vi "VSTest - Deploy and Run SLSC Module.vi"(8 "error in (no error)":errorcluster, 9 "Gateway IP Address":string="localhost", 10 "Slot Module Number":u32=3, 11 "SLSC Chassis IP Address":string="10.2.228.104") -> (0 "error out":errorcluster, 3 "Passed?":bool)   [LabVIEW 2015, in "SLSC EDS Testing.lvlib"]
uses:
  SLSC EDS Testing.lvlib
  <vilib>/Utility/sysdir.llb/System Directory Type.ctl
  <vilib>/NI Veristand/Execution/Workspace/NI VeriStand - Get Multiple Channel Values.vi
  <vilib>/NI Veristand/Execution/Workspace/NI_VS Workspace ExecutionAPI.lvlib
  SLSC UI API/SLSC Tree Control.lvlib
  SLSC EDS API/SLSC EDS API.lvlib
panel:
  out "Command to launch VS":string
  out "appended path":path
  out "State":string="Done!"
  out "Initial State Defined?":bool
  out "Dynamic Property Equal?":bool
  out "Measured Values":dbl[](array[numeric])=[3.0, 5.0]
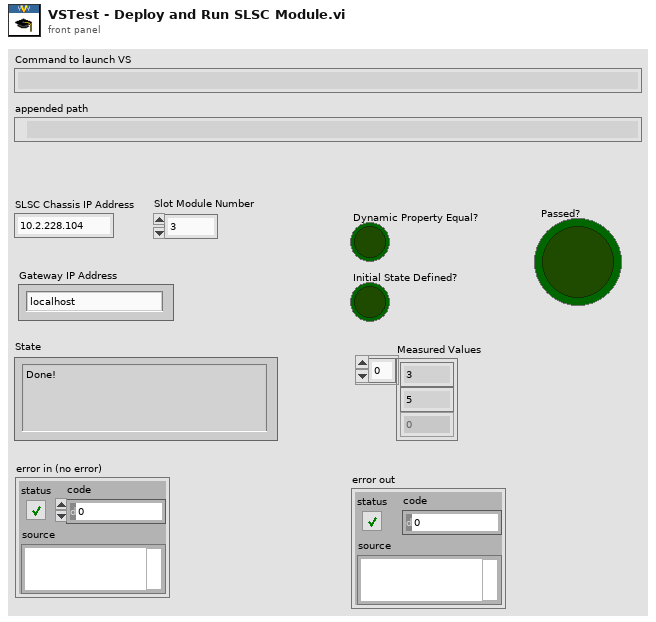
[diagram p1: front panel]
types:
  T1 = typedef "System Directory Type.ctl" = i32
  T2 = typedef "EDSjsonStructure.ctl" = cluster{"vendorNum":u32, "vendorName":string, "vendorPrefix":string, "productNum":u32, "productName":string, "capsVersion":string, "capsSpecVersion":u32, "capsSpecOldestCompatibleVersion":u32, "enums":T3[], "properties":T4[], "commands":T5[], "scales":T6[], "physicalChannels":T7[], "registerMap":cluster{"registers":T8[]}}
  T3 = typedef "enum.ctl" = cluster{"name":string, "description-en":string, "values":cluster{"name":string, "description-en":string, "value":i32}[]}
  T4 = typedef "property.ctl" = cluster{"name":string, "description-en":string, "documentation-en":string, "dataType":string, "bitfield":string, "access":string, "scale":string, "value":variant, "min":variant, "max":variant, "default value":variant}
  T5 = typedef "command.ctl" = cluster{"name":string, "description-en":string, "documentation-en":string, "startBitfield":string, "waitTimeInMs":i32, "doneBitfield":string, "doneInterrupt":string, "doneTimeoutInMs":i32, "value":variant}
  T6 = typedef "scale.ctl" = cluster{"name":string, "description-en":string, "m":dbl, "b":dbl, "forwardCoeffs":dbl[], "reverseCoeffs":dbl[], "coercion":string, "table":cluster{"scaled":dbl, "unscaled":dbl}[]}
  T7 = typedef "physicalChannel.ctl" = cluster{"name":string, "description-en":string, "commands":T5[], "properties":T4[]}
  T8 = typedef "register.ctl" = cluster{"name":string, "description-en":string, "access":string, "address":u32, "size":u32, "bitfields":cluster{"name":string, "description-en":string, "offset":u32, "size":u32, "signed":bool, "strobe":bool}[]}
  T9 = typedef "NI_VS Workspace ExecutionAPI.lvlib/WorkspaceAPI.ctl" = refnum<k24>
  T10 = cluster{"Left Cell String":string, "Child Text":string[], "Child Tag":string, "Item Indent":i32, "Child Only?":bool, "Glyph Index":i32}[]
  T11 = cluster{"Left Cell String":string, "Child Text":string[], "Child Tag":string, "Item Indent":i32, "Child Only?":bool, "Glyph Index":i32}
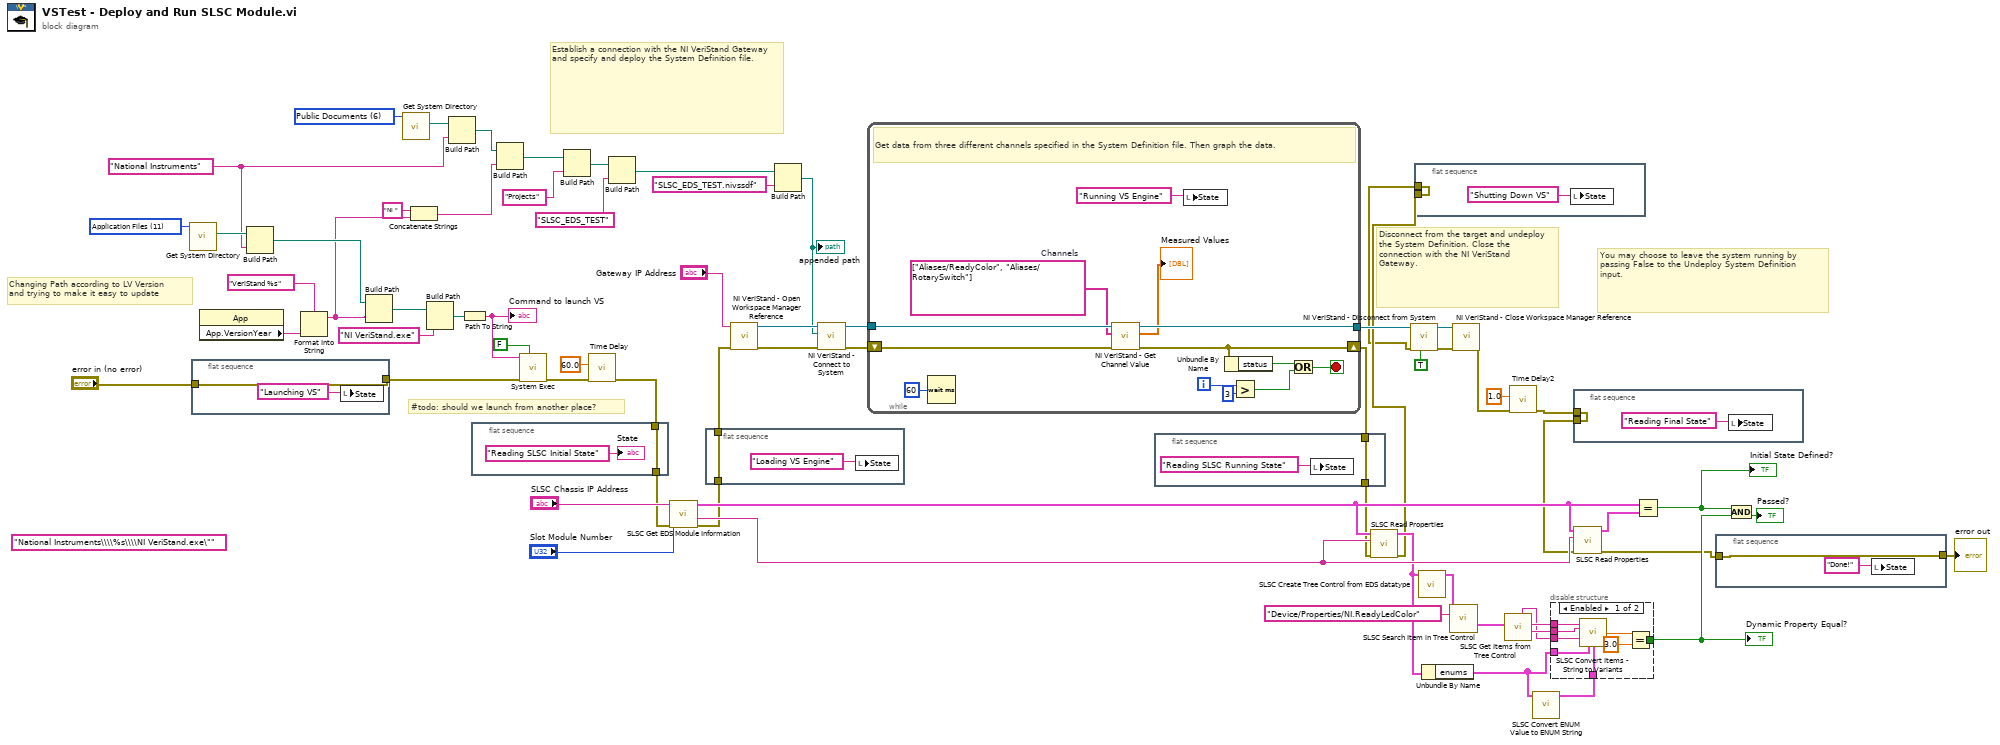
[diagram p0: block diagram]
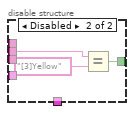
[diagram p2: hidden frame]
diagram:
  w15 = "National Instruments" ("command line")
  w20 = T1 11 items=["User Home"=0, "User Desktop"=1, "User Documents"=2, "User Application Data"=3, "User Preferences"=4, "User Temporary"=5, "Public Documents"=6, "Public Application Data"=7, "Public Preferences"=8, "Public Cache"=13, "System Core Libraries"=9, "System Installed Libraries"=10, "Application Files"=11, "Boot Volume Root"=12] ("system directory type")
  w21 = T1 6 items=["User Home"=0, "User Desktop"=1, "User Documents"=2, "User Application Data"=3, "User Preferences"=4, "User Temporary"=5, "Public Documents"=6, "Public Application Data"=7, "Public Preferences"=8, "Public Cache"=13, "System Core Libraries"=9, "System Installed Libraries"=10, "Application Files"=11, "Boot Volume Root"=12] ("system directory type")
  (unwired) "National Instruments\\\\%s\\\\NI VeriStand.exe\"" ("command line")
  # "Changing Path according to LV Version\nand trying to make it easy to update"
  # "#todo: should we launch from another place?"
  # "You may choose to leave the system running by passing False to the Undeploy System Definition input."
  # "Establish a connection with the NI VeriStand Gateway and specify and deploy the System Definition file."
  # "Disconnect from the target and undeploy the System Definition. Close the connection with the NI VeriStand Gateway."
  n1 = call <vilib>:"Get System Directory.vi"("system directory type"=w20) -> ("system directory"=w16:path)  [unwired: 10 in]
  n2 = flat-sequence {
    tunnel: "error in (no error)" -> [w69]
    tunnel: [w69] -> w23
    frame #0 {
      n3 = local write "State"("Launching VS" ("State")) -> ()
    }
  }
  n4 = property class="App"() -> ("App.VersionYear"=w22:string)  [unwired: 2 in, 2 out]
  n5 = Build Path(base path=w16, name or relative path=w15) -> (appended path=w14:path)
  n6 = Format Into String(format string="VeriStand %s" ("command line"), w22) -> (resulting string=w13:string)  [unwired: 2 in, 1 out]
  n7 = Build Path(base path=w14, name or relative path=w13) -> (appended path=w8:path)
  n8 = call <vilib>:"Get System Directory.vi"("system directory type"=w21) -> ("system directory"=w19:path)  [unwired: 10 in]
  n9 = Concatenate Strings("NI " ("string"), w13) -> (w3:string)
  n10 = Build Path(base path=w8, name or relative path="NI VeriStand.exe" ("command line")) -> (appended path=w7:path)
  n11 = Build Path(base path=w19, name or relative path=w15) -> (appended path=w17:path)
  n12 = Path To String(path=w7) -> (string=w10:string)
  "Command to launch VS" <- w10
  n13 = flat-sequence {
    tunnel: w35 -> [w71]
    tunnel: [w71] -> w34
    frame #0 {
      "State" <- "Reading SLSC Initial State" ("State")
    }
  }
  n14 = Build Path(base path=w17, name or relative path=w3) -> (appended path=w6:path)
  n15 = call <vilib>:"System Exec.vi"("wait until completion? (T)"=FALSE, "error in (no error)"=w23, "command line"=w10) -> ("error out"=w59:errorcluster)  [unwired: 5 in, 3 out]
  n16 = Build Path(base path=w6, name or relative path="Projects") -> (appended path=w5:path)
  n17 = call "Time Delay"("error in (no error)"=w59, "Delay Time (s)"=60.0) -> ("error out"=w35:errorcluster)  [unwired: 9 in]
  n18 = Build Path(base path=w5, name or relative path="SLSC_EDS_TEST") -> (appended path=w12:path)
  n19 = call "SLSC Get EDS Module Information.vi"("error in (no error)"=w34, "Slot #"="Slot Module Number", "Chassis IP Address"="SLSC Chassis IP Address") -> ("error out"=w33:errorcluster, "SLSC Module Name"=w41:string, "SLSC EDS module"=w42:T2)  [unwired: 5 in, 1 out]
  n20 = flat-sequence {
    tunnel: w33 -> [w73]
    tunnel: [w73] -> w32
    frame #0 {
      n21 = local write "State"("Loading VS Engine" ("State")) -> ()
    }
  }
  n22 = call <vilib>:"NI VeriStand - Open Workspace Manager Reference.vi"("error in (no error)"=w32, "Gateway IP Address (\"\": localhost)"="Gateway IP Address") -> ("error out"=w61:errorcluster, "WorkspaceManager"=w60:T9)  [unwired: 8 in]
  n23 = Build Path(base path=w12, name or relative path="SLSC_EDS_TEST.nivssdf") -> (appended path=w51:path)
  "appended path" <- w51
  n24 = call <vilib>:"NI VeriStand - Connect to System.vi"("error in (no error)"=w61, "System Definition File (.nivssdf)"=w51, "WorkspaceManager in"=w60) -> ("error out"=w64:errorcluster, "WorkspaceManager out"=w63:T9)  [unwired: 7 in]
  n25 = while {
    shift-right: [w84] -> w31
    shift-left: w64 -> [w85]
    tunnel: w63 -> [w83]
    tunnel: [w82] -> w62
    i -> [w78]
    stop <- w87 stop-if-true
    w80 = string[] ["Aliases/ReadyColor", "Aliases/RotarySwitch"]  # Channels
    # "Get data from three different channels specified in the System Definition file. Then graph the data."
    n26 = Wait (ms)(milliseconds to wait=u32 60) -> ()  [unwired: 1 out]
    n27 = call-poly <vilib>:"NI VeriStand - Get Channel Value.vi"("error in (no error)"=w85, "Channels"=w80, "WorkspaceManager in"=w83) -> ("error out"=w84:errorcluster, "Values"=→"Measured Values":dbl[], "WorkspaceManager out"=w82:T9)  [unwired: 6 in]
    n28 = local write "State"("Running VS Engine" ("State")) -> ()
    n29 = Unbundle By Name(w84) -> ("status"=w86:bool)
    n30 = Greater?(x=w78, y=3) -> (0:w76:bool)
    n31 = Or(x=w86, y=w76) -> (x .or. y?=w87:bool)
  }
  n32 = flat-sequence {
    tunnel: w31 -> [w88]
    tunnel: [w88] -> w30
    frame #0 {
      n33 = local write "State"("Reading SLSC Running State" ("State")) -> ()
    }
  }
  n34 = call "SLSC Read Properties.vi"("error in (no error)"=w30, "SLSC Device"=w41, "SLSC EDS module in"=w42) -> ("error out"=w29:errorcluster, "SLSC EDS module out"=w38:T2)  [unwired: 7 in]
  n35 = call <vilib>:"NI VeriStand - Disconnect from System.vi"("Undeploy System Definition (F)"=TRUE, "error in (no error)"=w28, "WorkspaceManager in"=w62) -> ("error out"=w67:errorcluster, "WorkspaceManager out"=w66:T9)  [unwired: 7 in]
  n36 = flat-sequence {
    tunnel: w29 -> [w90]
    tunnel: [w90] -> w28
    frame #0 {
      n37 = local write "State"("Shutting Down VS" ("State")) -> ()
    }
  }
  n38 = call "SLSC Create Tree Control from EDS datatype.vi"("SLSC EDS module"=w38) -> ("SLSC Output Tree"=w39:T10)  [unwired: 7 in, 3 out]
  n39 = Unbundle By Name(w38) -> ("enums"=w37:T3[])
  n40 = call "SLSC Search Item in Tree Control.vi"("SLSC Output Tree"=w39, "Item Tag"="Device/Properties/NI.ReadyLedColor") -> ("Item"=w46:T11)  [unwired: 10 in, 3 out]
  n41 = call <vilib>:"NI VeriStand - Close Workspace Manager Reference.vi"("error in (no error)"=w67, "WorkspaceManager"=w66) -> ("error out"=w55:errorcluster)  [unwired: 9 in]
  n42 = call "SLSC Get Items from Tree Control.vi"("Item"=w46) -> ("Value"=w44:string, "Datatype"=w45:string, "Reset Value"=w43:string)  [unwired: 6 in, 2 out]
  n43 = call "Time Delay2"("error in (no error)"=w55, "Delay Time (s)"=1.0) -> ("error out"=w26:errorcluster)  [unwired: 9 in]
  n44 = call "SLSC Convert ENUM Value to ENUM String.vi"("enums"=w37) -> ("string enums"=w36:cluster{"name":string, "string enums":string}[])  [unwired: 10 in]
  n45 = disable-structure shown="Enabled" {
    disable-tunnel: w45 -> [w99 _]
    disable-tunnel: w44 -> [w98 w101]
    disable-tunnel: w43 -> [w97 _]
    disable-tunnel: [w94 w102] -> w53
    disable-tunnel: w37 -> [w93 _]
    disable-tunnel: w36 -> [w92 _]
    frame Enabled {
      n46 = call "SLSC Convert Items - String to Variants.vi"("Datatype"=w99, "Value"=w98, "Reset Value"=w97, "enums"=w93, "string enums"=w92) -> ("Value (DBL)"=w96:dbl)  [unwired: 7 in, 3 out]
      n47 = Equal?(x=w96, y=3.0) -> (x = y?=w94:bool)
    }
    frame Disabled {
      n48 = Equal?(x=w101, y="[3]Yellow") -> (x = y?=w102:bool)
    }
  }
  "Dynamic Property Equal?" <- w53
  n49 = flat-sequence {
    tunnel: [w103] -> w27
    tunnel: w26 -> [w103]
    frame #0 {
      n50 = local write "State"("Reading Final State" ("State")) -> ()
    }
  }
  n51 = call "SLSC Read Properties.vi"("error in (no error)"=w27, "SLSC Device"=w41, "SLSC EDS module in"=w42) -> ("error out"=w25:errorcluster, "SLSC EDS module out"=w40:T2)  [unwired: 7 in]
  n52 = Equal?(x=w42, y=w40) -> (x = y?=w52:bool)
  "Initial State Defined?" <- w52
  n53 = flat-sequence {
    tunnel: [w105] -> w1
    tunnel: w25 -> [w105]
    frame #0 {
      n54 = local write "State"("Done!" ("State")) -> ()
    }
  }
  n55 = And(x=w52, y=w53) -> (x .and. y?=→"Passed?":bool)
  "error out" <- w1
